vi "old_HWGlobalsToCols.vi"(7 "Select Layout":refnum<vi>, 8 "error in (no error)":errorcluster, 9 "SetList Display":bool[](array[boolean]), 10 "Column Names":string[](array[string]), 11 "Device in":refnum<class "Device.lvclass">) -> (0 "error out":errorcluster, 3 "Device out":refnum<class "Device.lvclass">)   [LabVIEW 2013, in "Device.lvclass"]
doc: "Write Column Names and SetList Display (optional \"compressed\" view layout from RbI) to Device columns. If SetList Display is not empty, a \"Legacy\" layout is appended to the Select Layout ring, unless it already exists."
uses:
  Device.lvclass
  ColumnVIs/Column/Column.lvclass
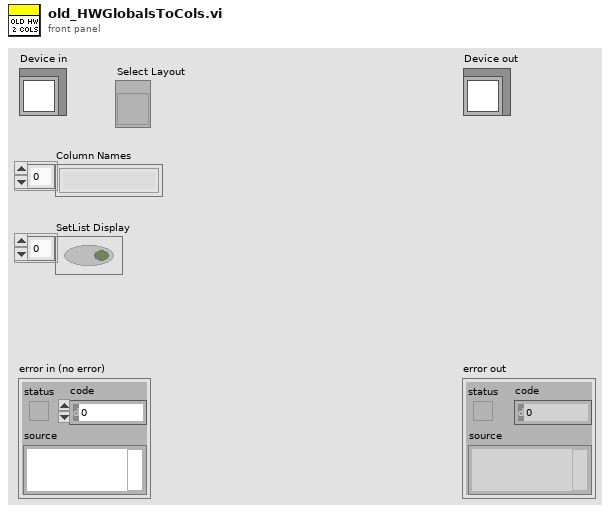
[diagram p1: front panel]
types:
  T1 = typedef "ColumnAppearCluster.ctl" = cluster{"Column Name":string, "Width":u32, "Bkgd":u32[], "Text":u32[]}
  T2 = typedef "LVStringsAndValuesArrayTypeDef_I32.ctl" = cluster{"String":string, "Value":i32}[]
  T3 = typedef "ColumnLayoutCluster.ctl" = cluster{"Label":string, "Color":u32, "Width":u32, "[disp?]":bool[]}
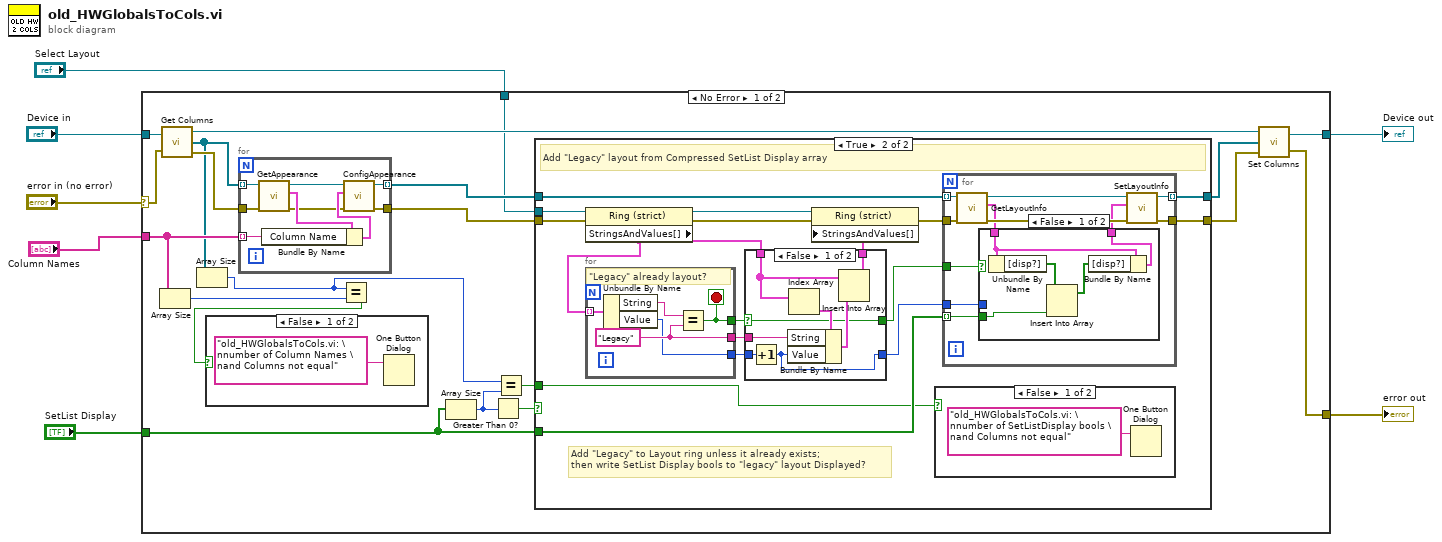
[diagram p0: block diagram]
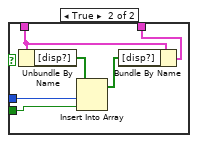
[diagram p4: hidden frame]
diagram:
  n1 = case shown="No Error" "error in (no error)" {
    selector: "error in (no error)" -> [w23 w97]
    tunnel: [w22 w97] -> w6
    tunnel: [w24 w96] -> w4
    tunnel: "Device in" -> [w25 w96]
    tunnel: "Column Names" -> [w21 _]
    tunnel: "SetList Display" -> [w16 _]
    tunnel: "Select Layout" -> [w11 _]
    frame No Error {
      n2 = Array Size(array=w21) -> (size(s)=w20:i32)
      n3 = call-dynamic "Get Columns.vi"("Device in"=w25, "error in (no error)"=w23) -> ("Device out"=w26:refnum<class "Device.lvclass">, "Columns"=w9:refnum<class "Column.lvclass">[], "error out"=w27:errorcluster)
      n4 = Array Size(array=w9) -> (size(s)=w8:i32)
      n5 = for {
        tunnel: w9 -> [w91] mode=indexing
        tunnel: [w90] -> w18 mode=indexing
        tunnel: w27 -> [w89]
        tunnel: [w88] -> w17
        tunnel: w21 -> [w87] mode=indexing
        n6 = call "GetAppearance.vi"("error in (no error)"=w89, "Column in"=w91) -> ("error out"=w92:errorcluster, "Column Appearance"=w94:T1, "Column out"=w95:refnum<class "Column.lvclass">)  [unwired: 7 in]
        n7 = Bundle By Name(cluster=w94, "Column Name"=w87) -> (w93:T1)
        n8 = call "ConfigAppearance.vi"("error in (no error)"=w92, "Column Appearance"=w93, "Column in"=w95) -> ("error out"=w88:errorcluster, "Column out"=w90:refnum<class "Column.lvclass">)  [unwired: 7 in]
      }
      n9 = Equal?(x=w8, y=w20) -> (x = y?=w19:bool)
      n10 = case shown="False" w19 {
        frame False {
          n11 = One Button Dialog(message="old_HWGlobalsToCols.vi: \nnumber of Column Names \nand Columns not equal") -> ()  [unwired: 1 in, 1 out]
        }
        frame True {
        }
      }
      n12 = Array Size(array=w16) -> (size(s)=w10:i32)
      n13 = Greater Than 0?(x=w10) -> (x > 0?=w15:bool)
      n14 = Equal?(x=w8, y=w10) -> (x = y?=w12:bool)
      n15 = case shown="True" w15 {
        tunnel: w18 -> [w29 w37]
        tunnel: w17 -> [w28 w38]
        tunnel: w16 -> [_ w33]
        tunnel: [w29 w36] -> w14
        tunnel: [w28 w34] -> w13
        tunnel: w12 -> [_ w32]
        tunnel: w11 -> [_ w46]
        frame False {
          # "With an empty SetList Display input, the device will have a \"default shown\" appearance\nfor all existing items in Select Layout."
          # "No \"legacy\" view provided."
        }
        frame True {
          # "Add \"Legacy\" to Layout ring unless it already exists;\nthen write SetList Display bools to \"legacy\" layout Displayed?"
          # "Add \"Legacy\" layout from Compressed SetList Display array"
          n16 = property class="Ring (strict)"(reference=w46, error in=w38) -> (reference out=w44:refnum<vi>, error out=w45:errorcluster, "StringsAndValues[]"=w42:T2)
          n17 = for {
            tunnel: w42 -> [w85] mode=indexing
            tunnel: [w81] -> w40
            tunnel: [w83] -> w41
            tunnel: [w82] -> w39
            stop <- w82 stop-if-true
            w83 = "Legacy"
            # "\"Legacy\" already layout?"
            n18 = Unbundle By Name(w85) -> ("String"=w84:string, "Value"=w81:i32)
            n19 = Equal?(x=w84, y=w83) -> (x = y?=w82:bool)
          }
          n20 = case shown="False" w39 {
            selector: w39 -> [w70 w78]
            tunnel: [w77 w80] -> w43
            tunnel: w42 -> [w74 w80]
            tunnel: w41 -> [w73 _]
            tunnel: w40 -> [w72 w79]
            tunnel: [w71 w79] -> w30
            tunnel: [w70 w78] -> w31
            frame False {
              n21 = Increment(x=w72) -> (x+1=w71:i32)
              n22 = Index Array(array=w74) -> (element=w76:cluster{"String":string, "Value":i32})  [unwired: 1 in]
              n23 = Bundle By Name(cluster=w76, "String"=w73, "Value"=w71) -> (w75:cluster{"String":string, "Value":i32})
              n24 = Insert Into Array(array=w74, new element=w75) -> (w77:T2)  [unwired: 1 in]
            }
            frame True {
            }
          }
          n25 = property class="Ring (strict)"(reference=w44, error in=w45, "StringsAndValues[]"=w43) -> (error out=w35:errorcluster)  [unwired: 1 out]
          n26 = case shown="False" w32 {
            frame False {
              n27 = One Button Dialog(message="old_HWGlobalsToCols.vi: \nnumber of SetListDisplay bools \nand Columns not equal") -> ()  [unwired: 1 in, 1 out]
            }
            frame True {
            }
          }
          n28 = for {
            tunnel: w37 -> [w56] mode=indexing
            tunnel: w35 -> [w55]
            tunnel: w33 -> [w50] mode=indexing
            tunnel: [w54] -> w36 mode=indexing
            tunnel: [w53] -> w34
            tunnel: w31 -> [w52]
            tunnel: w30 -> [w49]
            n29 = call "GetLayoutInfo.vi"("error in (no error)"=w55, "Column in"=w56) -> ("error out"=w58:errorcluster, "Layout cluster"=w51:T3, "Column out"=w57:refnum<class "Column.lvclass">)  [unwired: 7 in]
            n30 = case shown="False" w52 {
              tunnel: [w63 w69] -> w48
              tunnel: w51 -> [w62 w68]
              tunnel: w50 -> [w60 w66]
              tunnel: w49 -> [_ w65]
              frame False {
                n31 = Unbundle By Name(w62) -> ("[disp?]"=w61:bool[])
                n32 = Insert Into Array(array=w61, new element=w60) -> (w59:bool[])  [unwired: 1 in]
                n33 = Bundle By Name(cluster=w62, "[disp?]"=w59) -> (w63:T3)
              }
              frame True {
                n34 = Unbundle By Name(w68) -> ("[disp?]"=w67:bool[])
                n35 = Insert Into Array(array=w67, index=w65, new element=w66) -> (w64:bool[])
                n36 = Bundle By Name(cluster=w68, "[disp?]"=w64) -> (w69:T3)
              }
            }
            n37 = call "SetLayoutInfo.vi"("error in (no error)"=w58, "Layout cluster"=w48, "Column in"=w57) -> ("error out"=w53:errorcluster, "Column out"=w54:refnum<class "Column.lvclass">)  [unwired: 7 in]
          }
        }
      }
      n38 = call-dynamic "Set Columns.vi"("error in (no error)"=w13, "Columns"=w14, "Device in"=w26) -> ("error out"=w22:errorcluster, "Device out"=w24:refnum<class "Device.lvclass">)  [unwired: 1 in]
    }
    frame Error {
    }
  }
  "error out" <- w6
  "Device out" <- w4
